vi "Map2D.vi"() -> ()   [LabVIEW 2023]
panel:
  out "Map element":map{string, i32}(c390)
  in  "On index":i32
  out "Array Of Maps":map{string, i32}[](array[numeric])
  out "2D Double Array":i32[][](array[numeric])
  out "Number":u64
  out "map out":map{string, i32}(c390)
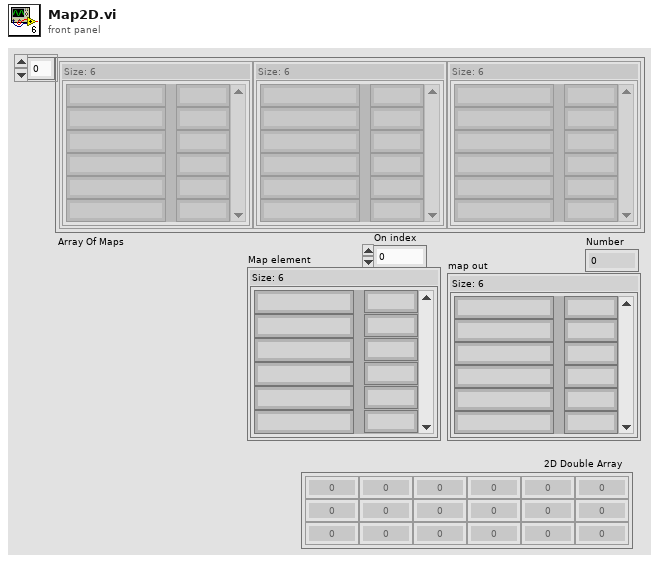
[diagram p1: front panel]
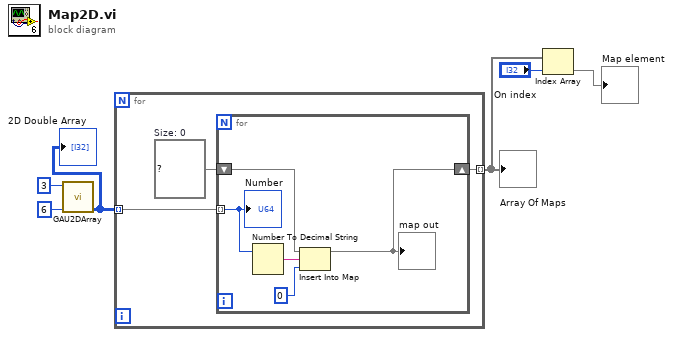
[diagram p0: block diagram]
diagram:
  n1 = call "GAU2DArray.vi"("Colums"=6 ("Colum"), "Rows"=3 ("Row")) -> ("2D Double Array"=w4:i32[][])  [unwired: 8 in, 1 out]
  "2D Double Array" <- w4
  n2 = for {
    tunnel: w4 -> [w9] mode=indexing
    tunnel: [w7] -> w3 mode=indexing
    w8 = map{string, i32} {}  # Size: 0
    n3 = for {
      tunnel: w9 -> [w12] mode=indexing
      shift-right: [w14] -> w7
      shift-left: w8 -> [w13]
      n4 = Number To Decimal String(number=w12) -> (decimal integer string=w11:string)  [unwired: 1 in]
      n5 = Insert Into Map(map in=w13, key=w11, value=0) -> (map out=w14:map{string, i32})  [unwired: 2 out]
      "map out" <- w14
      "Number" <- w12
    }
  }
  "Array Of Maps" <- w3
  n6 = Index Array "Index Array"(array=w3, index="On index") -> (element=→"Map element":map{string, i32})
